vi "Stop Core.vi"(10 "final error code":i32, 11 "1600 Card Actor in":refnum<class "1600 Card Actor.lvclass">) -> (3 "1600 Card Actor out":refnum<class "1600 Card Actor.lvclass">)   [LabVIEW 2012, in "Universal Power Meter.lvlib" / "WT1600.lvlib" / "1600Card.lvlib" / "1600 Card Actor.lvclass"]
doc: "(<B>Filename</B>: Actor Framework.lvlib:Actor.lvclass:Stop Core.vi)\n\nDefines what the actor does before it stops. Use the <B>final error code</B> input to determine whether the actor shut down in response to an error.\n\nBy default, this method does nothing. A descendant class may override it to define behavior, such as shutting down any processes the actor initiated in its override of the Actor Core method."
uses:
  1600 Card Actor.lvclass
  Observer Pattern Actor Template/Observer/Observer.lvclass
  <vilib>/ActorFramework/Actor/Actor.lvclass/Actor.ctl
  <vilib>/ActorFramework/Message Enqueuer/Message Enqueuer.lvclass/Message Enqueuer.ctl
  1600 Card Actor.lvclass/1600 Card Actor.ctl
  Observer Pattern Actor Template/Subject Messages/Remove Observer Msg/Remove Observer Msg.lvclass/Remove Observer Msg.ctl
  WT1600/WT1600 Messages/Cluster write one Msg/Cluster write one Msg.lvclass/Cluster write one Msg.ctl
  <vilib>/ActorFramework/Stop Msg/Stop Msg.lvclass/Stop Msg.ctl
  <vilib>/ActorFramework/Message Enqueuer/Init from Existing Queue.vi
  <vilib>/ActorFramework/Message Enqueuer/Enqueue.vi
  <vilib>/ActorFramework/Stop Msg/Send Emergency Stop.vi
  <vilib>/ActorFramework/Stop Msg/Send Normal Stop.vi
  <vilib>/ActorFramework/Message Enqueuer/Enqueue Critical.vi
  <vilib>/ActorFramework/Message Priority Queue/Priority Enqueue.vi
  <vilib>/ActorFramework/Message Enqueuer/Message Enqueuer.lvclass
  Observer Pattern Actor Template/Subject Messages/Remove Observer Msg/Remove Observer Msg.lvclass
  WT1600/WT1600 Messages/Cluster write one Msg/Cluster write one Msg.lvclass
  <vilib>/ActorFramework/Stop Msg/Stop Msg.lvclass
  <vilib>/ActorFramework/Actor/Actor.lvclass
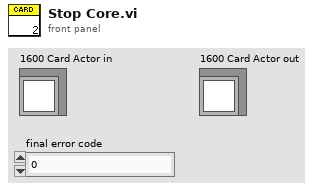
[diagram p1: front panel]
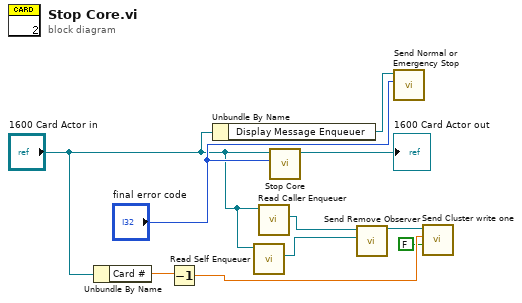
[diagram p0: block diagram]
diagram:
  n1 = Unbundle By Name("1600 Card Actor in") -> ("Card #"=w3:dbl)
  n2 = Decrement(x=w3) -> (x-1=w2:dbl)
  n3 = Unbundle By Name("1600 Card Actor in") -> ("Display Message Enqueuer"=w9:refnum<class "Message Enqueuer.lvclass">)
  n4 = call <vilib>:"Read Self Enqueuer.vi"("Actor"="1600 Card Actor in") -> ("Self Enqueuer"=w6:refnum<class "Message Enqueuer.lvclass">)  [unwired: 10 in]
  n5 = call <vilib>:"Read Caller Enqueuer.vi"("Actor"="1600 Card Actor in") -> ("Caller Enqueuer"=w7:refnum<class "Message Enqueuer.lvclass">)  [unwired: 10 in]
  n6 = call-parent "Stop Core.vi"("final error code"="final error code", "Actor in"="1600 Card Actor in") -> ("Actor out"=→"1600 Card Actor out":refnum<class "1600 Card Actor.lvclass">)  [unwired: 9 in]
  n7 = call "Send Remove Observer.vi"("Observer"=w6, "Message Enqueuer"=w7) -> ("Message Enqueuer out"=w5:refnum<class "Message Enqueuer.lvclass">)  [unwired: 8 in, 1 out]
  n8 = call <vilib>:"Send Normal or Emergency Stop.vi"("final error code"="final error code", "Message Enqueuer"=w9) -> ()  [unwired: 9 in, 1 out]
  n9 = call "Send Cluster write one.vi"("new element/subarray"=FALSE, "index of cluster"=w2, "Message Enqueuer"=w5) -> ()  [unwired: 7 in, 2 out]
